vi "SelectErrorControlType.vi"(1 "Error control type (primary)":T1, 12 "Error control type (secondary)":T1) -> (21 "Error control path":path)   [LabVIEW 2017, in "ErrorStructureDrawer.lvlib"]
doc: "Gets a path to the error control that corresponds to the type specified by \"Error control type (primary)\".\n\nIf the specified type is \"LabVIEW default\", then this VI will attempt to read the LabVIEW INI file to find out what the default type is. If that fails, or if the default type is not supported, then the VI will use the type specified by \"Error control type (secondary)\".\n\nIf the secondary choice is also \"LabVIEW default\", then the Modern type will be used."
uses:
  ErrorStructureDrawer.lvlib
  Controls/ErrorControlType.ctl
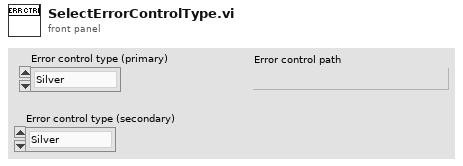
[diagram p1: front panel]
types:
  T1 = typedef "ErrorStructureDrawer.lvlib/ErrorControlType.ctl" = enum16{"Silver", "Modern", "Classic", "LabVIEW default", "NXG"}
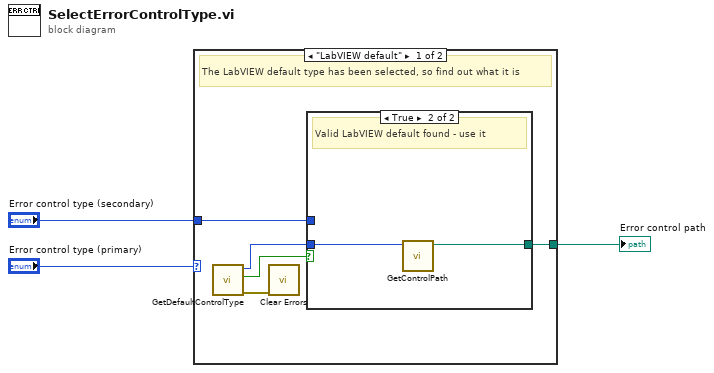
[diagram p0: block diagram]
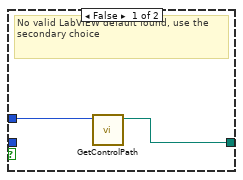
[diagram p2: hidden frame]
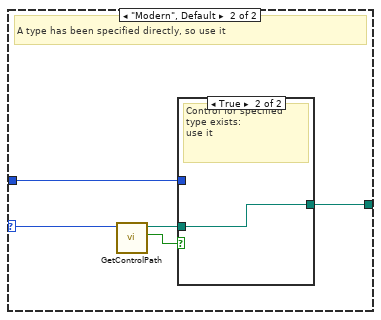
[diagram p3: hidden frame]
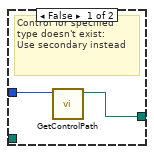
[diagram p4: hidden frame]
diagram:
  n1 = case shown="\"LabVIEW default\"" "Error control type (primary)" {
    selector: "Error control type (primary)" -> [_ w15]
    tunnel: [w4 w16] -> w1
    tunnel: "Error control type (secondary)" -> [w5 w14]
    frame "LabVIEW default" {
      # "The LabVIEW default type has been selected, so find out what it is"
      n2 = call "GetDefaultControlType.vi"() -> ("Error Out"=w8:errorcluster, "Default control style valid?"=w7:bool, "Error control type"=w6:T1)  [unwired: 9 in]
      n3 = call <vilib>:"Clear Errors.vi"("error in (no error)"=w8) -> ()  [unwired: 5 in, 2 out]
      n4 = case shown="True" w7 {
        tunnel: w6 -> [_ w12]
        tunnel: w5 -> [w10 _]
        tunnel: [w9 w11] -> w4
        frame False {
          # "No valid LabVIEW default found, use the secondary choice"
          n5 = call "GetControlPath.vi"("Error control type"=w10) -> ("Path"=w9:path)  [unwired: 9 in, 1 out]
        }
        frame True {
          # "Valid LabVIEW default found - use it"
          n6 = call "GetControlPath.vi"("Error control type"=w12) -> ("Path"=w11:path)  [unwired: 9 in, 1 out]
        }
      }
    }
    frame "Modern", Default {
      # "A type has been specified directly, so use it"
      n7 = call "GetControlPath.vi"("Error control type"=w15) -> ("Exists?"=w17:bool, "Path"=w13:path)  [unwired: 9 in]
      n8 = case shown="True" w17 {
        tunnel: [w18 w20] -> w16
        tunnel: w14 -> [w19 _]
        tunnel: w13 -> [_ w20]
        frame False {
          # "Control for specified type doesn't exist:\nUse secondary instead"
          n9 = call "GetControlPath.vi"("Error control type"=w19) -> ("Path"=w18:path)  [unwired: 9 in, 1 out]
        }
        frame True {
          # "Control for specified type exists:\nuse it"
        }
      }
    }
  }
  "Error control path" <- w1
